vi "getSelectionValuesLength.vi"(8 "error in (no error)":errorcluster, 11 "IProperty in":refnum<class "IProperty.lvclass">) -> (0 "error out":errorcluster, 1 "Selection Values Null?":bool, 2 "List.Size":i32, 3 "Dict.Size":i32, 4 "List?":bool, 5 "Dict?":bool)   [LabVIEW 2022 SP3, in "Property Editor.lvlib"]
uses:
  <instrlib>/openDAQ/Examples/Property Editor/Property Editor.lvlib
  <instrlib>/openDAQ/Public/Classes/IProperty/IProperty.lvclass
  <instrlib>/openDAQ/Public/Classes/IBaseObject/Polymorphic/borrowInterface/borrowListInterface.vi
  <instrlib>/openDAQ/Public/Classes/daqCoreTypes/IList/Polymorphic/getList/getBoolList.vi
  <instrlib>/openDAQ/Public/Classes/daqCoreTypes/IList/Polymorphic/getList/getIntegerList.vi
  <instrlib>/openDAQ/Public/Classes/daqCoreTypes/IList/Polymorphic/getList/getFloatList.vi
  <instrlib>/openDAQ/Public/Classes/daqCoreTypes/IList/Polymorphic/getList/getStringList.vi
  <instrlib>/openDAQ/Public/Classes/daqCoreTypes/IList/Polymorphic/getList/getRatioList.vi
  <instrlib>/openDAQ/Public/Classes/daqCoreTypes/IList/Polymorphic/getList/getProcedureList.vi
  <instrlib>/openDAQ/Public/Classes/daqCoreTypes/IList/Polymorphic/getList/getBaseObjectList.vi
  <instrlib>/openDAQ/Public/Classes/daqCoreTypes/IList/Polymorphic/getList/getFunctionList.vi
  <instrlib>/openDAQ/Public/Classes/daqCoreTypes/IList/Polymorphic/getList/getComplexNumberList.vi
  <instrlib>/openDAQ/Public/Classes/daqCoreTypes/IList/Polymorphic/getList/getStructList.vi
  <instrlib>/openDAQ/Public/Classes/daqCoreTypes/IList/Polymorphic/getList/getEnumerationList.vi
  <instrlib>/openDAQ/Public/Classes/IBaseObject/Polymorphic/borrowInterface/borrowDictInterface.vi
  <instrlib>/openDAQ/Public/Classes/daqCoreTypes/IDict/Polymorphic/getKeyList/getIntKeyList.vi
  <instrlib>/openDAQ/Public/Classes/IBaseObject/IBaseObject.lvclass
  <instrlib>/openDAQ/Public/Classes/daqCoreTypes/IDict/IDict.lvclass
  <instrlib>/openDAQ/Public/Classes/daqCoreTypes/IList/IList.lvclass
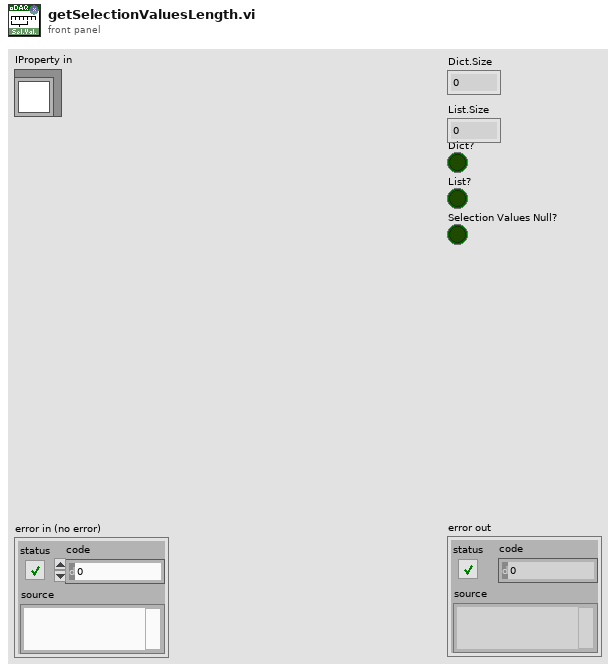
[diagram p1: front panel]
types:
  T1 = typedef "openDAQ.lvlib/CoreType.ctl" = u16
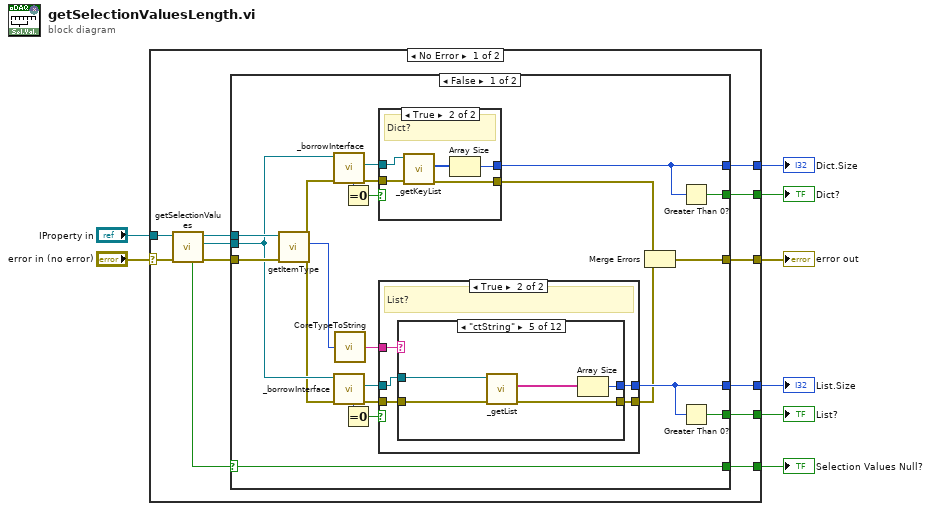
[diagram p0: block diagram]
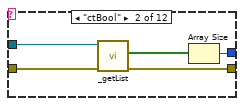
[diagram p4: hidden frame]
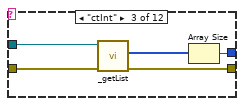
[diagram p5: hidden frame]
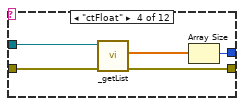
[diagram p6: hidden frame]
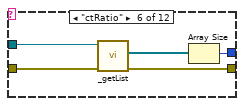
[diagram p7: hidden frame]
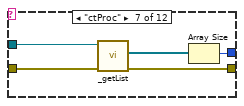
[diagram p8: hidden frame]
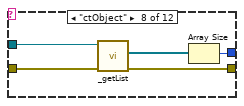
[diagram p9: hidden frame]
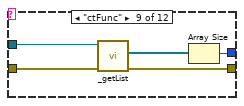
[diagram p10: hidden frame]
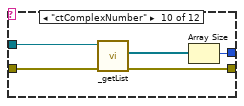
[diagram p11: hidden frame]
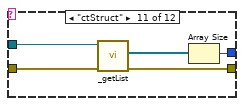
[diagram p12: hidden frame]
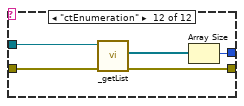
[diagram p13: hidden frame]
diagram:
  n1 = case shown="No Error" "error in (no error)" {
    selector: "error in (no error)" -> [w19 w113]
    tunnel: [w9 w113] -> w7
    tunnel: "IProperty in" -> [w20 _]
    tunnel: [w11 _] -> w1
    tunnel: [w16 _] -> w5
    tunnel: [w15 _] -> w4
    tunnel: [w14 _] -> w3
    tunnel: [w13 _] -> w2
    frame No Error {
      n2 = call <instrlib>:"getSelectionValues.vi"("error in (no error)"=w19, "IProperty in"=w20) -> ("error out"=w17:errorcluster, "Selection Values out"=w10:refnum<class "IBaseObject.lvclass">, "IProperty out"=w18:refnum<class "IProperty.lvclass">, "Null?"=w12:bool)  [unwired: 6 in]
      n3 = case shown="False" w12 {
        selector: w12 -> [w21 w111]
        tunnel: w18 -> [w42 _]
        tunnel: w17 -> [w41 w112]
        tunnel: w10 -> [w40 _]
        tunnel: [w28 _] -> w16
        tunnel: [w27 _] -> w15
        tunnel: [w26 _] -> w14
        tunnel: [w25 _] -> w13
        tunnel: [w22 w112] -> w9
        tunnel: [w21 w111] -> w11
        frame False {
          n4 = call <instrlib>:"getItemType.vi"("error in (no error)"=w41, "IProperty in"=w42) -> ("error out"=w29:errorcluster, "Item Type out"=w32:T1)  [unwired: 7 in, 1 out]
          n5 = call-poly <instrlib>:"_borrowInterface.vi"("error in (no error)"=w29, "IBaseObject in"=w40) -> ("error out"=w36:errorcluster, "Dict out"=w35:refnum<class "IDict.lvclass">, "err"=w39:u32)  [unwired: 6 in, 1 out]
          n6 = call-poly <instrlib>:"_borrowInterface.vi"("error in (no error)"=w29, "IBaseObject in"=w40) -> ("error out"=w34:errorcluster, "List out"=w33:refnum<class "IList.lvclass">, "err"=w38:u32)  [unwired: 6 in, 1 out]
          n7 = call <instrlib>:"CoreTypeToString.vi"("Value Type out"=w32) -> ("String"=w31:string)  [unwired: 4 in]
          n8 = Equal To 0?(x=w39) -> (x = 0?=w37:bool)
          n9 = Equal To 0?(x=w38) -> (x = 0?=w30:bool)
          n10 = case shown="True" w37 {
            tunnel: w36 -> [w105 w109]
            tunnel: w35 -> [_ w110]
            tunnel: [_ w107] -> w28
            tunnel: [w105 w106] -> w23
            frame False {
            }
            frame True {
              # "Dict?"
              n11 = call-poly <instrlib>:"_getKeyList.vi"("error in (no error)"=w109, "IDict in"=w110) -> ("error out"=w106:errorcluster, "Key List out"=w108:i32[])  [unwired: 7 in, 1 out]
              n12 = Array Size(array=w108) -> (size(s)=w107:i32)
            }
          }
          n13 = case shown="True" w30 {
            tunnel: w34 -> [w43 w47]
            tunnel: w33 -> [_ w46]
            tunnel: w31 -> [_ w48]
            tunnel: [_ w45] -> w26
            tunnel: [w43 w44] -> w24
            frame False {
            }
            frame True {
              # "List?"
              n14 = case shown="\"ctString\"" w48 {
                tunnel: w47 -> [w49 w54 w59 w64 w69 w74 w79 w84 w89 w94 w99 w104]
                tunnel: w46 -> [_ w53 w58 w63 w68 w73 w78 w83 w88 w93 w98 w103]
                tunnel: [_ w51 w56 w61 w66 w71 w76 w81 w86 w91 w96 w101] -> w45
                tunnel: [w49 w50 w55 w60 w65 w70 w75 w80 w85 w90 w95 w100] -> w44
                frame Default {
                }
                frame "ctBool" {
                  n15 = call-poly <instrlib>:"_getList.vi"("error in (no error)"=w54, "IList in"=w53) -> ("error out"=w50:errorcluster, "Booleans out"=w52:bool[])  [unwired: 8 in]
                  n16 = Array Size(array=w52) -> (size(s)=w51:i32)
                }
                frame "ctInt" {
                  n17 = call-poly <instrlib>:"_getList.vi"("error in (no error)"=w59, "IList in"=w58) -> ("error out"=w55:errorcluster, "Integers out"=w57:i32[])  [unwired: 8 in]
                  n18 = Array Size(array=w57) -> (size(s)=w56:i32)
                }
                frame "ctFloat" {
                  n19 = call-poly <instrlib>:"_getList.vi"("error in (no error)"=w64, "IList in"=w63) -> ("error out"=w60:errorcluster, "Floats out"=w62:dbl[])  [unwired: 8 in]
                  n20 = Array Size(array=w62) -> (size(s)=w61:i32)
                }
                frame "ctString" {
                  n21 = call-poly <instrlib>:"_getList.vi"("error in (no error)"=w69, "IList in"=w68) -> ("error out"=w65:errorcluster, "String List out"=w67:string[])  [unwired: 8 in]
                  n22 = Array Size(array=w67) -> (size(s)=w66:i32)
                }
                frame "ctRatio" {
                  n23 = call-poly <instrlib>:"_getList.vi"("error in (no error)"=w74, "IList in"=w73) -> ("error out"=w70:errorcluster, "Ratios out"=w72:refnum<class "IRatio.lvclass">[])  [unwired: 8 in]
                  n24 = Array Size(array=w72) -> (size(s)=w71:i32)
                }
                frame "ctProc" {
                  n25 = call-poly <instrlib>:"_getList.vi"("error in (no error)"=w79, "IList in"=w78) -> ("error out"=w75:errorcluster, "devices out"=w77:refnum<class "IProcedure.lvclass">[])  [unwired: 8 in]
                  n26 = Array Size(array=w77) -> (size(s)=w76:i32)
                }
                frame "ctObject" {
                  n27 = call-poly <instrlib>:"_getList.vi"("error in (no error)"=w84, "IList in"=w83) -> ("error out"=w80:errorcluster, "baseObjects out"=w82:refnum<class "IBaseObject.lvclass">[])  [unwired: 8 in]
                  n28 = Array Size(array=w82) -> (size(s)=w81:i32)
                }
                frame "ctFunc" {
                  n29 = call-poly <instrlib>:"_getList.vi"("error in (no error)"=w89, "IList in"=w88) -> ("error out"=w85:errorcluster, "devices out"=w87:refnum<class "IFunction.lvclass">[])  [unwired: 8 in]
                  n30 = Array Size(array=w87) -> (size(s)=w86:i32)
                }
                frame "ctComplexNumber" {
                  n31 = call-poly <instrlib>:"_getList.vi"("error in (no error)"=w94, "IList in"=w93) -> ("error out"=w90:errorcluster, "devices out"=w92:refnum<class "IComplexNumber.lvclass">[])  [unwired: 8 in]
                  n32 = Array Size(array=w92) -> (size(s)=w91:i32)
                }
                frame "ctStruct" {
                  n33 = call-poly <instrlib>:"_getList.vi"("error in (no error)"=w99, "IList in"=w98) -> ("error out"=w95:errorcluster, "devices out"=w97:refnum<class "IStruct.lvclass">[])  [unwired: 8 in]
                  n34 = Array Size(array=w97) -> (size(s)=w96:i32)
                }
                frame "ctEnumeration" {
                  n35 = call-poly <instrlib>:"_getList.vi"("error in (no error)"=w104, "IList in"=w103) -> ("error out"=w100:errorcluster, "devices out"=w102:refnum<class "IEnumeration.lvclass">[])  [unwired: 8 in]
                  n36 = Array Size(array=w102) -> (size(s)=w101:i32)
                }
              }
            }
          }
          n37 = Merge Errors(w23, w24) -> (w22:errorcluster)
          n38 = Greater Than 0?(x=w28) -> (x > 0?=w27:bool)
          n39 = Greater Than 0?(x=w26) -> (x > 0?=w25:bool)
        }
        frame True {
        }
      }
    }
    frame Error {
    }
  }
  "error out" <- w7
  "Dict.Size" <- w5
  "Dict?" <- w4
  "List.Size" <- w3
  "List?" <- w2
  "Selection Values Null?" <- w1
